vi "Set ICommunicate.vi"(10 "ICommunicate":refnum<class "ICommunicate.lvclass">, 11 "CANopen Master in":refnum<class "CANopen Master.lvclass">) -> (3 "CANopen Master out":refnum<class "CANopen Master.lvclass">)   [LabVIEW 2024, in "CANopen Master.lvlib" / "CANopen Master.lvclass"]
uses:
  CANopen Master.lvclass
  HAL/Source/Interfaces/ICommunicate/ICommunicate.lvclass
  CANopen Master.lvclass/CANopen Master.ctl
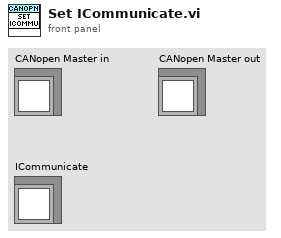
[diagram p1: front panel]
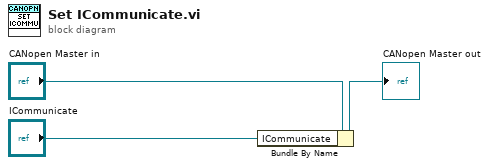
[diagram p0: block diagram]
diagram:
  n1 = Bundle By Name(cluster="CANopen Master in", "ICommunicate"="ICommunicate") -> (→"CANopen Master out":refnum<class "CANopen Master.lvclass">)
